vi "EmergencyStop.vi"(0 "object in":refnum<class "Logger.lvclass">, 2 "Emergency":bool, 5 "error in (no error)":errorcluster) -> (14 "object out":refnum<class "Logger.lvclass">, 19 "error out":errorcluster)   [LabVIEW 2014, in "Logger.lvclass"]
uses:
  Logger.lvclass
  Logger.lvclass/Logger.ctl
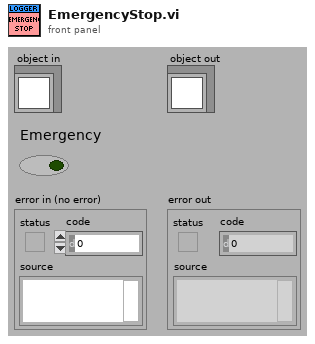
[diagram p1: front panel]
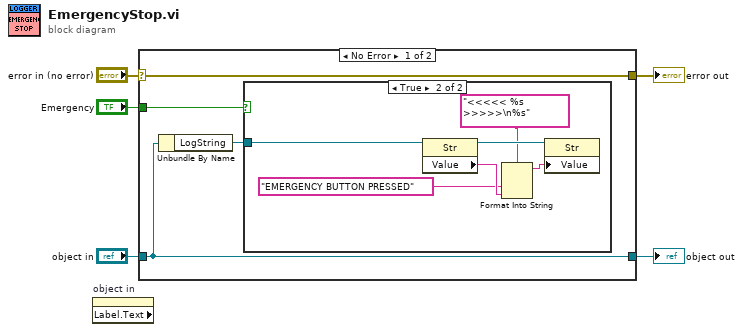
[diagram p0: block diagram]
diagram:
  n1 = property on="object in" class="LVClassControl (strict)" props=["Label", "Text"]() -> ()  [unwired: 2 in, 3 out]
  n2 = case shown="No Error" "error in (no error)" {
    selector: "error in (no error)" -> [w9 w17]
    tunnel: [w9 w17] -> w4
    tunnel: [w7 w16] -> w2
    tunnel: "object in" -> [w7 w16]
    tunnel: "Emergency" -> [w6 _]
    frame No Error {
      n3 = Unbundle By Name(w7) -> ("LogString"=w8:refnum<vi>)
      n4 = case shown="True" w6 {
        tunnel: w8 -> [_ w14]
        frame False {
        }
        frame True {
          n5 = property class="Str"(reference=w14) -> (reference out=w15:refnum<vi>, "Value"=w13:string)  [unwired: 1 in, 1 out]
          n6 = Format Into String(format string="<<<<< %s >>>>>\n%s", "EMERGENCY BUTTON PRESSED" ("input 1"), w13) -> (resulting string=w12:string)  [unwired: 2 in, 1 out]
          n7 = property class="Str"(reference=w15, "Value"=w12) -> ()  [unwired: 1 in, 2 out]
        }
      }
    }
    frame Error {
    }
  }
  "error out" <- w4
  "object out" <- w2
